vi "Run_VI.vi"(0 "Application_Directory":path, 11 "Error_In":errorcluster) -> (15 "Error_Out":errorcluster)   [LabVIEW 2023]
doc: "Used to run a vi."
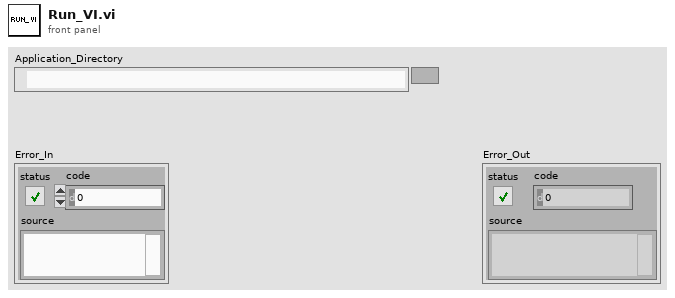
[diagram p1: front panel]
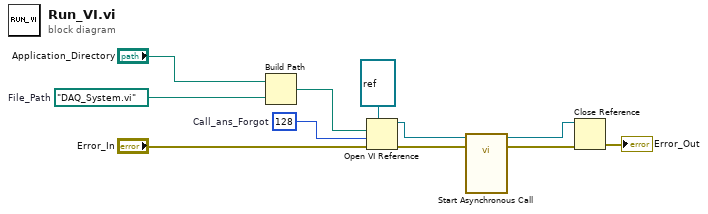
[diagram p0: block diagram]
diagram:
  w8 = 128  # Call_ans_Forgot
  w9 = path "DAQ_System.vi"  # File_Path
  n1 = Build Path(base path="Application_Directory", name or relative path=w9) -> (appended path=w10:path)
  n2 = Open VI Reference(type specifier VI Refnum (for type only)=refnum<vi> refnum, vi path=w10, options=w8, error in (no error)="Error_In") -> (vi reference=w5:refnum<vi>, error out=w7:errorcluster)  [unwired: 2 in]
  n3 = call-by-ref "Start Asynchronous Call"(reference=w5, error in=w7) -> (reference out=w4:refnum<vi>, error out=w6:errorcluster)  [unwired: 16 in]
  n4 = Close Reference(reference=w4, error in (no error)=w6) -> (error out=→"Error_Out":errorcluster)
